vi "Manual Driver Test.vi"() -> ()   [LabVIEW 2020, in "polar_bear_plus_drivers.lvlib"]
uses:
  <instrlib>/RxnRover/Driver Polar Bear Plus/polar_bear_plus_drivers.lvlib
  <instrlib>/RxnRover/Driver Polar Bear Plus/heater_parent/heater_parent.lvclass
  <instrlib>/RxnRover/Driver Polar Bear Plus/heater_explorer/heater_explorer.lvclass
  <instrlib>/RxnRover/Driver Polar Bear Plus/heater_flow_synthesiser/heater_flow_synthesiser.lvclass
  C:/Program Files (x86)/National Instruments/LabVIEW 2020/instr.lib/RxnRover/Polar Bear Plus All-in-One/heater_parent/heater_parent.lvclass
panel:
  in  "Get Current Temperature Btn":bool
  out "Current Temperature":dbl
  in  "Start Heating Btn":bool
  in  "Stop Heating Btn":bool
  in  "Change Temperature Setpoint":dbl
  in  "Set Temperature Setpoint Btn":bool
  in  "Get Temperature Setpoint Btn":bool
  out "Current Temperature Setpoint":dbl
  in  "stop":bool
  out "Max Temperature":dbl
  in  "Get Max Temperature Btn":bool
  in  "Close Driver Btn":bool
  in  "Initialization Options":T1={"Select a Driver"="heater_explorer", "Initialize Driver Btn"=FALSE, "Reset (False)"=FALSE, "Modbus Address"=255, "IP Address"="147.155.248.82", "Data File Directory"=path "C:/Program Files (x86)/National Instruments/LabVIEW 2020/instr.lib/Eurotherm nanodac/Public/Utility/nanodac V4_20"}
  out "error out":errorcluster
  in  "error in (no error)":errorcluster
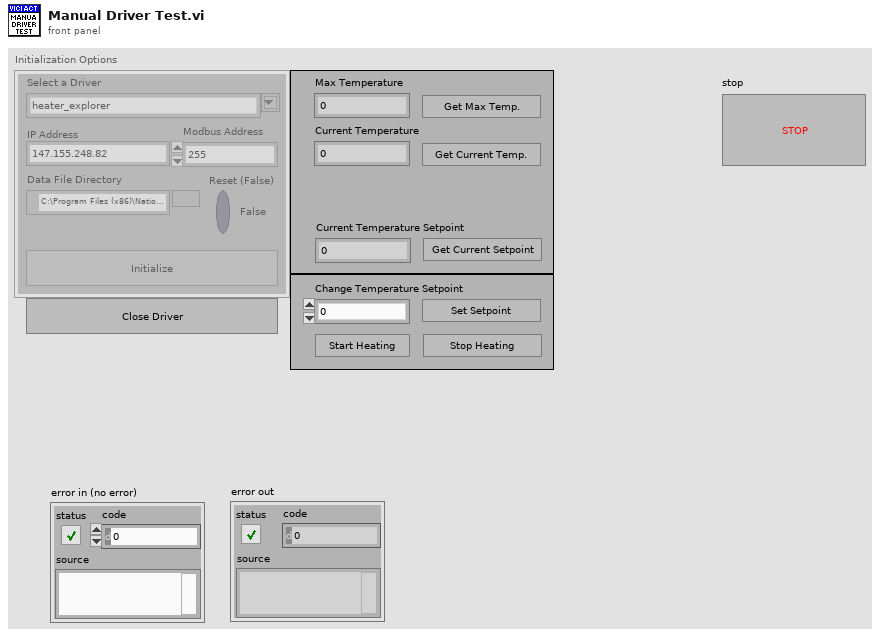
[diagram p1: front panel]
types:
  T1 = cluster{"Select a Driver":string, "Initialize Driver Btn":bool, "Reset (False)":bool, "Modbus Address":u8, "IP Address":string, "Data File Directory":path}
  T2 = enum8{"Enabled", "Disabled", "Disabled and Grayed Out"}
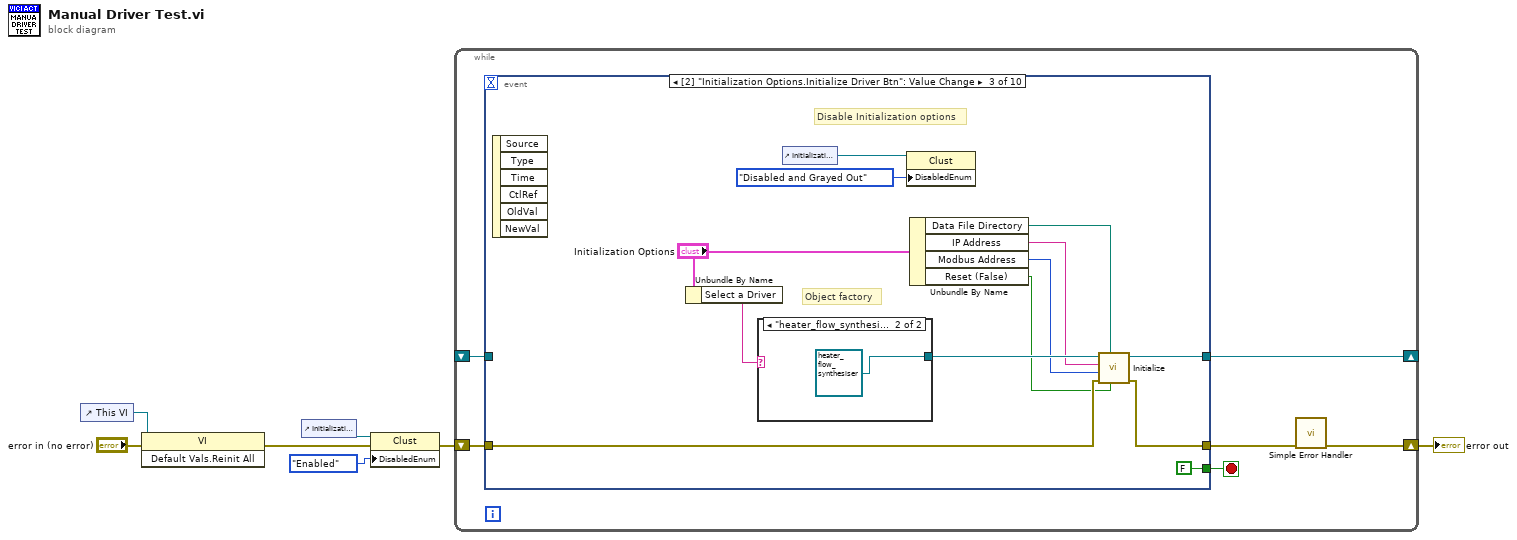
[diagram p0: block diagram]
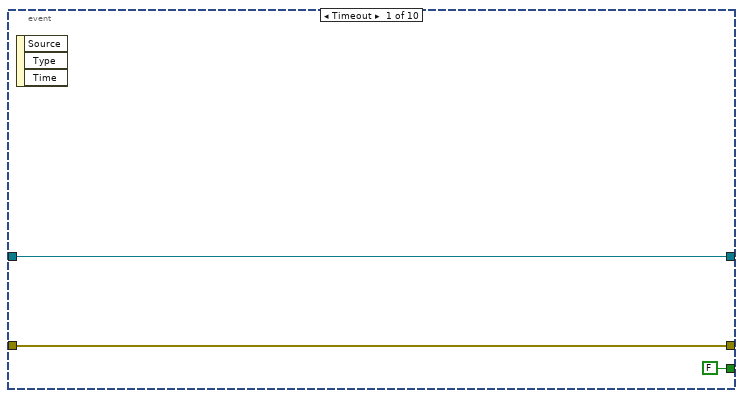
[diagram p2: hidden frame]
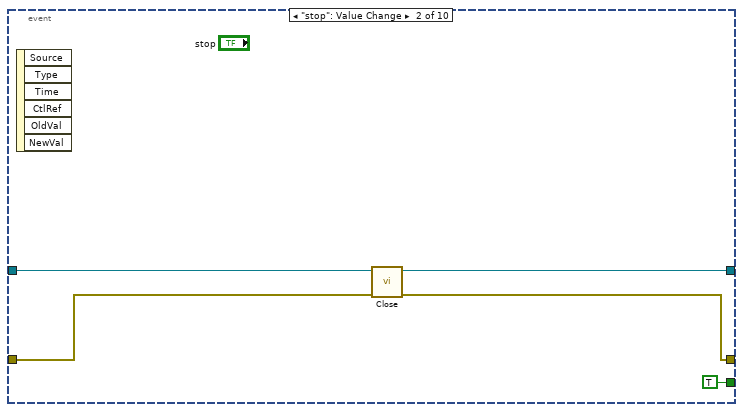
[diagram p3: hidden frame]
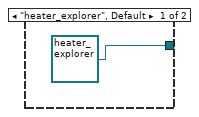
[diagram p4: hidden frame]
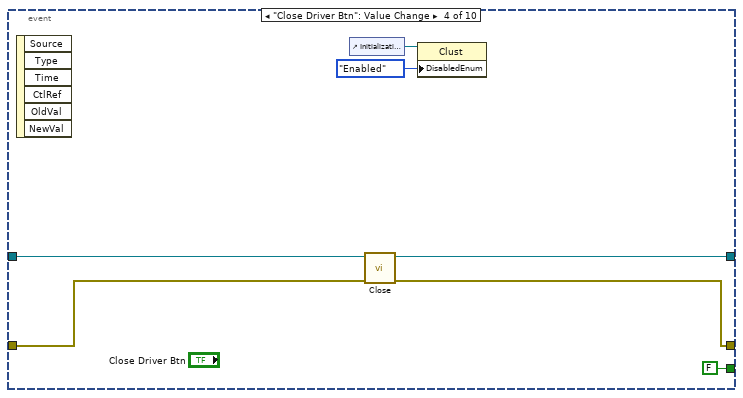
[diagram p5: hidden frame]
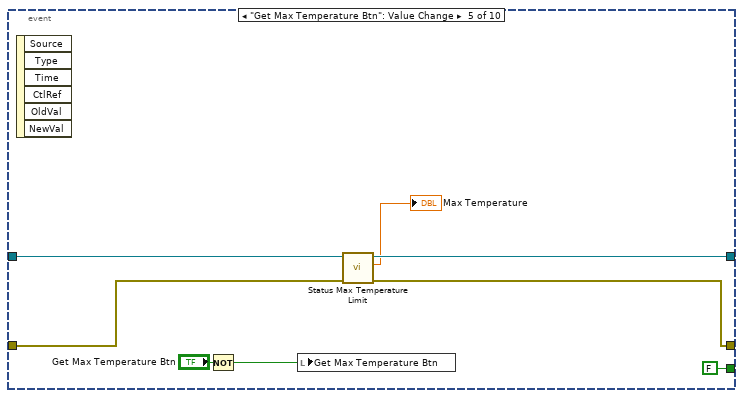
[diagram p6: hidden frame]
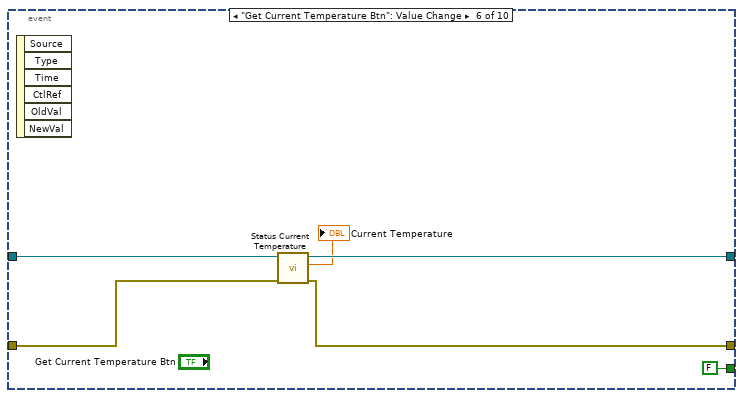
[diagram p7: hidden frame]
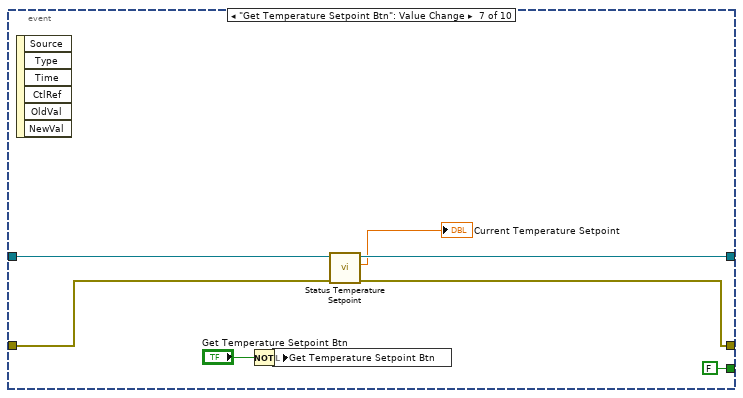
[diagram p8: hidden frame]
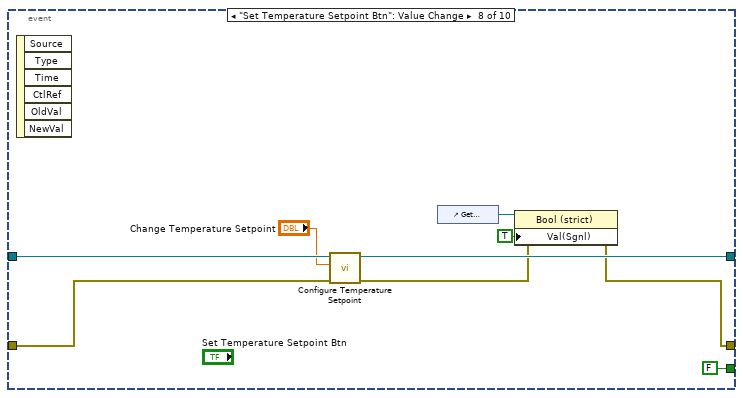
[diagram p9: hidden frame]
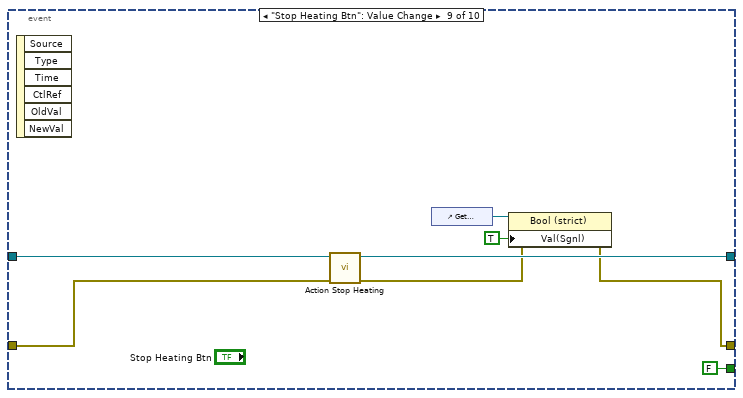
[diagram p10: hidden frame]
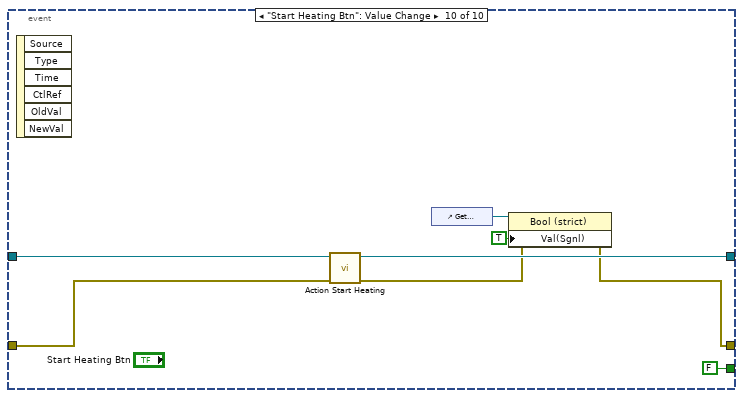
[diagram p11: hidden frame]
diagram:
  n1 = control-ref of="This VI"() -> (w1:refnum<vi>)
  n2 = invoke class="VI" method="Default Vals.Reinit All"(reference=w1, error in="error in (no error)") -> (error out=w2:errorcluster)  [unwired: 1 in, 2 out]
  n3 = control-ref of="Initialization Options"() -> (w6:refnum<vi>)
  n4 = property class="Clust"(reference=w6, error in=w2, "DisabledEnum"=T2."Enabled" ("Disabled")) -> (error out=w5:errorcluster)  [unwired: 1 out]
  n5 = while {
    shift-right: [w13] -> _
    shift-left: _ -> [w12]
    shift-right: [w8] -> w3
    shift-left: w5 -> [w11]
    stop <- w9 stop-if-true
    n6 = event shown="[2] \"Initialization Options.Initialize Driver Btn\": Value Change" {
      selector: _ -> [_ _ _ _ _ _ _ _ _ _]
      dyn-events: _ -> [_ _ _ _ _ _ _ _ _ _]
      timeout: _ -> [_ _ _ _ _ _ _ _ _ _]
      tunnel: [w14 w19 w29 w42 w48 w55 w63 w72 w80 w88] -> w13
      tunnel: w12 -> [w14 w20 _ w43 w51 w57 w64 w73 w81 w89]
      tunnel: w11 -> [w15 w17 w27 w41 w50 w56 w62 w71 w79 w87]
      tunnel: [w15 w18 w28 w40 w49 w52 w61 w67 w76 w83] -> w10
      tunnel: [FALSE TRUE FALSE FALSE FALSE FALSE FALSE FALSE FALSE FALSE] -> w9
      event Timeout {
        n7 = event-data() -> ()  [unwired: 1 in, 3 out]
      }
      event "stop": Value Change {
        n8 = event-data() -> ()  [unwired: 1 in, 6 out]
        n9 = call-dynamic "Close.vi"("error in (no error)"=w17, "heater_parent in"=w20) -> ("error out"=w18:errorcluster, "heater_parent out"=w19:refnum<class "heater_parent.lvclass">)  [unwired: 8 in]
      }
      event "Initialization Options.Initialize Driver Btn": Value Change {
        # "Disable Initialization options"
        # "Object factory"
        n10 = event-data() -> ()  [unwired: 1 in, 6 out]
        n11 = Unbundle By Name("Initialization Options") -> ("Select a Driver"=w32:string)
        n12 = case shown="\"heater_flow_synthesiser\"" w32 {
          tunnel: [refnum<class "heater_explorer.lvclass"> refnum ("polar_bear_plus_drivers.lvlib:heater_explorer.lvclass") refnum<class "heater_flow_synthesiser.lvclass"> refnum ("polar_bear_plus_drivers.lvlib:heater_flow_synthesiser.lvclass")] -> w26
          frame "heater_explorer", Default {
          }
          frame "heater_flow_synthesiser" {
          }
        }
        n13 = control-ref of="Initialization Options"() -> (w33:refnum<vi>)
        n14 = property class="Clust"(reference=w33, "DisabledEnum"=T2."Disabled and Grayed Out" ("Disabled")) -> ()  [unwired: 1 in, 2 out]
        n15 = Unbundle By Name("Initialization Options") -> ("Data File Directory"=w22:path, "IP Address"=w24:string, "Modbus Address"=w25:u8, "Reset (False)"=w23:bool)
        n16 = call-dynamic "Initialize.vi"("Reset (False)"=w23, "start path"=w22, "error in (no error)"=w27, "Modbus Address"=w25, "IP Address"=w24, "vici_flow_actuator_parent in"=w26) -> ("error out"=w28:errorcluster, "vici_flow_actuator_parent out"=w29:refnum<class "heater_parent.lvclass">)  [unwired: 3 in, 1 out]
      }
      event "Close Driver Btn": Value Change {
        n17 = event-data() -> ()  [unwired: 1 in, 6 out]
        n18 = control-ref of="Initialization Options"() -> (w38:refnum<vi>)
        n19 = call-dynamic "Close.vi"("error in (no error)"=w41, "heater_parent in"=w43) -> ("error out"=w40:errorcluster, "heater_parent out"=w42:refnum<class "heater_parent.lvclass">)  [unwired: 8 in]
        n20 = property class="Clust"(reference=w38, "DisabledEnum"=T2."Enabled" ("Disabled")) -> ()  [unwired: 1 in, 2 out]
      }
      event "Get Max Temperature Btn": Value Change {
        n21 = event-data() -> ()  [unwired: 1 in, 6 out]
        n22 = Not(x="Get Max Temperature Btn") -> (.not. x?=w44:bool)
        n23 = local write "Get Max Temperature Btn"(w44) -> ()
        n24 = call-dynamic "Status Max Temperature Limit.vi"("error in (no error)"=w50, "heater_parent in"=w51) -> ("error out"=w49:errorcluster, "Max Temperature Limit"=→"Max Temperature":dbl, "heater_parent out"=w48:refnum<class "heater_parent.lvclass">)  [unwired: 7 in]
      }
      event "Get Current Temperature Btn": Value Change {
        n25 = event-data() -> ()  [unwired: 1 in, 6 out]
        n26 = call-dynamic "Status Current Temperature.vi"("error in (no error)"=w56, "heater_parent in"=w57) -> ("error out"=w52:errorcluster, "Current Temperature"=→"Current Temperature":dbl, "heater_parent out"=w55:refnum<class "heater_parent.lvclass">)  [unwired: 7 in]
      }
      event "Get Temperature Setpoint Btn": Value Change {
        n27 = event-data() -> ()  [unwired: 1 in, 6 out]
        n28 = Not(x="Get Temperature Setpoint Btn") -> (.not. x?=w58:bool)
        n29 = local write "Get Temperature Setpoint Btn"(w58) -> ()
        n30 = call-dynamic "Status Temperature Setpoint.vi"("error in (no error)"=w62, "heater_parent in"=w64) -> ("error out"=w61:errorcluster, "Setpoint"=→"Current Temperature Setpoint":dbl, "heater_parent out"=w63:refnum<class "heater_parent.lvclass">)  [unwired: 7 in]
      }
      event "Set Temperature Setpoint Btn": Value Change {
        n31 = event-data() -> ()  [unwired: 1 in, 6 out]
        n32 = call-dynamic "Configure Temperature Setpoint.vi"("error in (no error)"=w71, "New Setpoint"="Change Temperature Setpoint", "heater_parent in"=w73) -> ("error out"=w68:errorcluster, "heater_parent out"=w72:refnum<class "heater_parent.lvclass">)  [unwired: 7 in]
        n33 = control-ref of="Get Temperature Setpoint Btn"() -> (w69:refnum<vi>)
        n34 = property class="Bool (strict)"(reference=w69, error in=w68, "Val(Sgnl)"=TRUE) -> (error out=w67:errorcluster)  [unwired: 1 out]
      }
      event "Stop Heating Btn": Value Change {
        n35 = event-data() -> ()  [unwired: 1 in, 6 out]
        n36 = call-dynamic "Action Stop Heating.vi"("error in (no error)"=w79, "heater_parent in"=w81) -> ("error out"=w77:errorcluster, "heater_parent out"=w80:refnum<class "heater_parent.lvclass">)  [unwired: 8 in]
        n37 = control-ref of="Get Temperature Setpoint Btn"() -> (w78:refnum<vi>)
        n38 = property class="Bool (strict)"(reference=w78, error in=w77, "Val(Sgnl)"=TRUE ("Value (Signaling)")) -> (error out=w76:errorcluster)  [unwired: 1 out]
      }
      event "Start Heating Btn": Value Change {
        n39 = event-data() -> ()  [unwired: 1 in, 6 out]
        n40 = call-dynamic "Action Start Heating.vi"("error in (no error)"=w87, "heater_parent in"=w89) -> ("error out"=w84:errorcluster, "heater_parent out"=w88:refnum<class "heater_parent.lvclass">)  [unwired: 8 in]
        n41 = control-ref of="Get Temperature Setpoint Btn"() -> (w86:refnum<vi>)
        n42 = property class="Bool (strict)"(reference=w86, error in=w84, "Val(Sgnl)"=TRUE) -> (error out=w83:errorcluster)  [unwired: 1 out]
      }
    }
    n43 = call <vilib>:"Simple Error Handler.vi"("error in (no error)"=w10) -> ("error out"=w8:errorcluster)  [unwired: 4 in, 4 out]
  }
  "error out" <- w3
